vi "Running VIs.vi"() -> ()   [LabVIEW 2020]
panel:
  out "Running 2":string[](array[string])
  out "Top Level":string[](array[string])
  out "Running":string[](array[string])
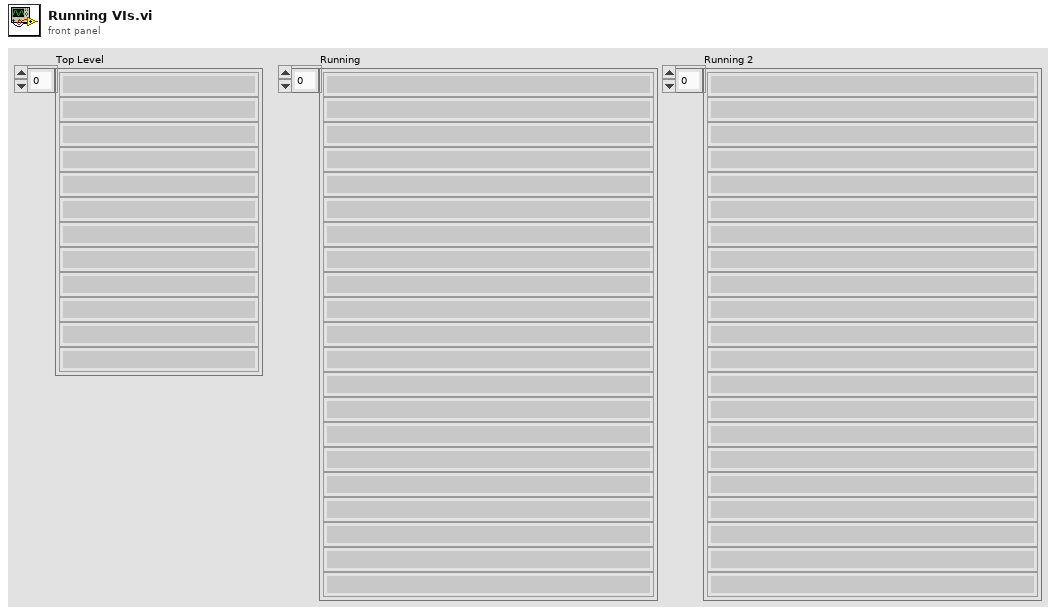
[diagram p1: front panel]
types:
  T1 = enum32{"Bad", "Idle", "Run top level", "Running"}
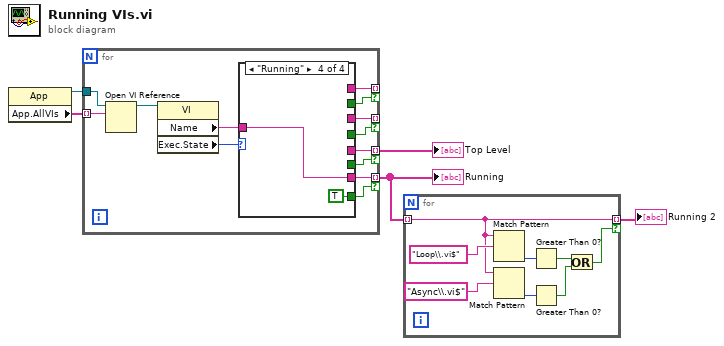
[diagram p0: block diagram]
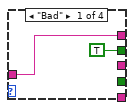
[diagram p2: hidden frame]
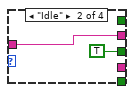
[diagram p3: hidden frame]
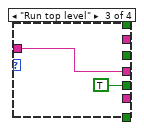
[diagram p4: hidden frame]
diagram:
  n1 = property class="App"() -> (reference out=w4:refnum<vi>, "App.AllVIs"=w5:string[])  [unwired: 2 in, 1 out]
  n2 = for {
    tunnel: w5 -> [w18] mode=indexing
    tunnel: w4 -> [w17]
    tunnel: [w14] -> _ mode=indexing if=w12
    tunnel: [w11] -> _ mode=indexing if=w10
    tunnel: [w9] -> w3 mode=indexing if=w8
    tunnel: [w7] -> w2 mode=indexing if=w6
    n3 = Open VI Reference(application reference (local)=w17, vi path=w18) -> (vi reference=w16:refnum<vi>)  [unwired: 4 in, 1 out]
    n4 = property class="VI"(reference=w16) -> ("Name"=w13:string, "Exec.State"=w15:T1)  [unwired: 1 in, 2 out]
    n5 = case shown="\"Running\"" w15 {
      tunnel: [w20 _ _ _] -> w14
      tunnel: w13 -> [w20 w22 w24 w26]
      tunnel: [TRUE _ _ _] -> w12
      tunnel: [_ w22 _ _] -> w11
      tunnel: [_ TRUE _ _] -> w10
      tunnel: [_ _ w24 _] -> w9
      tunnel: [_ _ TRUE _] -> w8
      tunnel: [_ _ _ w26] -> w7
      tunnel: [_ _ _ TRUE] -> w6
      frame "Bad" {
      }
      frame "Idle" {
      }
      frame "Run top level" {
      }
      frame "Running" {
      }
    }
  }
  "Running" <- w2
  "Top Level" <- w3
  n6 = for {
    tunnel: w2 -> [w30] mode=indexing
    tunnel: [w30] -> w1 mode=indexing if=w27
    n7 = Match Pattern(string=w30, regular expression="Loop\\.vi$") -> (offset past match=w32:i32)  [unwired: 1 in, 3 out]
    n8 = Match Pattern(string=w30, regular expression="Async\\.vi$") -> (offset past match=w31:i32)  [unwired: 1 in, 3 out]
    n9 = Greater Than 0?(x=w32) -> (x > 0?=w29:bool)
    n10 = Greater Than 0?(x=w31) -> (x > 0?=w28:bool)
    n11 = Or(x=w29, y=w28) -> (x .or. y?=w27:bool)
  }
  "Running 2" <- w1
